vi "Read input.vi"(8 "error in (no error)":errorcluster, 10 "Input":i32) -> (0 "error out":errorcluster, 2 "State":bool)   [LabVIEW 2022 SP3]
doc: "Reads input state\n-iologix E1210"
uses:
  <vilib>/NI/Modbus Library/API/Master/Modbus Master.lvclass
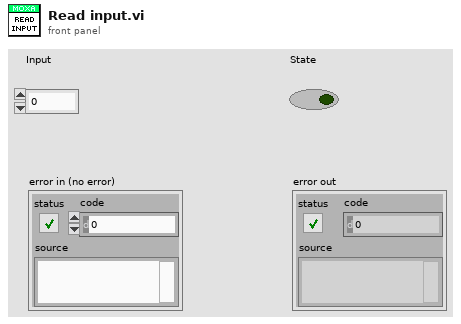
[diagram p1: front panel]
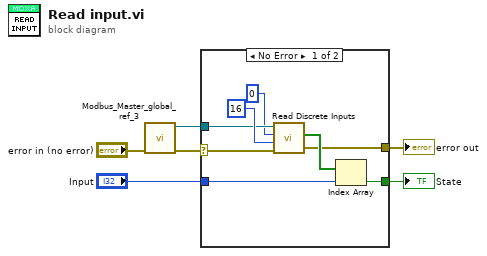
[diagram p0: block diagram]
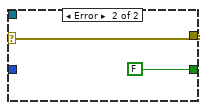
[diagram p2: hidden frame]
diagram:
  n1 = call "Modbus_Master_global_ref_3.vi"("error in (no error) 2"="error in (no error)") -> ("error out 2"=w1:errorcluster, "Modbus Master out"=w3:refnum<class "Modbus Master.lvclass">)  [unwired: 9 in]
  n2 = case shown="No Error" w1 {
    selector: w1 -> [w9 w16]
    tunnel: [w14 FALSE ("Boolean")] -> w6
    tunnel: "Input" -> [w7 _]
    tunnel: [w12 w16] -> w4
    tunnel: w3 -> [w10 _]
    frame No Error {
      n3 = call-dynamic "Read Discrete Inputs.vi"("error in"=w9, "number of inputs"=u16 16, "starting address"=u16 0, "Modbus master in"=w10) -> ("error out"=w12:errorcluster, "discrete inputs"=w13:bool[])  [unwired: 5 in, 1 out]
      n4 = Index Array(array=w13, index=w7) -> (element=w14:bool)
    }
    frame Error {
    }
  }
  "State" <- w6
  "error out" <- w4
